vi "checkCycleComplete.vi"(8 "error in (no error)":errorcluster, 11 "TestMonitor in":refnum<class "TestMonitor.lvclass">) -> (0 "error out":errorcluster, 2 "cycleCompleteIsTrue":bool, 3 "TestMonitor out":refnum<class "TestMonitor.lvclass">)   [LabVIEW 2015]
uses:
  TestMonitor.lvclass
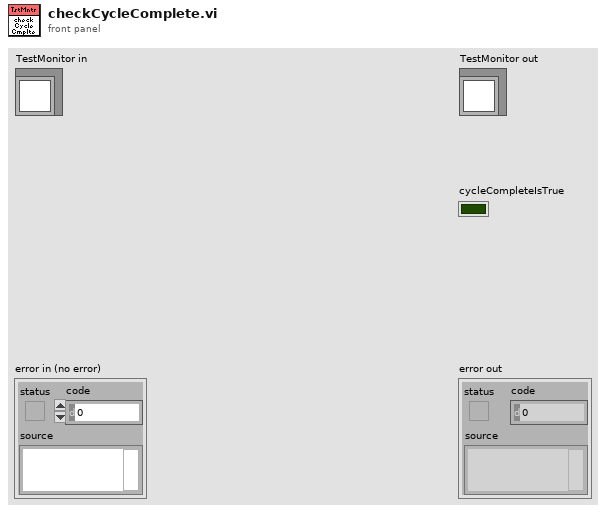
[diagram p1: front panel]
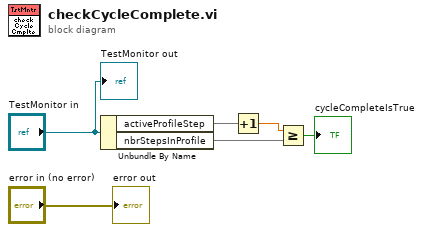
[diagram p0: block diagram]
diagram:
  n1 = Unbundle By Name("TestMonitor in") -> ("activeProfileStep"=w2, "nbrStepsInProfile"=w1)
  n2 = Increment(x=w2) -> (x+1=w3:dbl)
  n3 = Greater Or Equal?(x=w3, y=w1) -> (x >= y?=→"cycleCompleteIsTrue":bool)
  "error out" <- "error in (no error)"
  "TestMonitor out" <- "TestMonitor in"
